vi "StartCANEngine.vi"(8 "error in (no error)":errorcluster, 10 "Buses":string[](array[string]), 11 "SmartBench in":refnum<class "SmartBench.lvclass">) -> (0 "error out":errorcluster, 3 "SmartBench out":refnum<class "SmartBench.lvclass">)   [LabVIEW 2024, in "SmartBench.lvclass"]
uses:
  SmartBench.lvclass
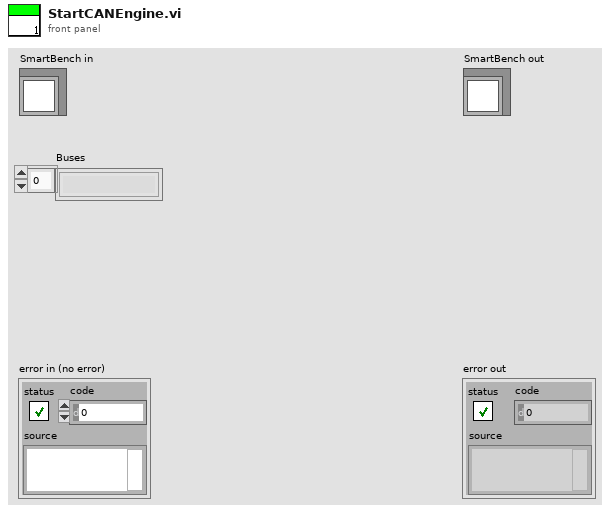
[diagram p1: front panel]
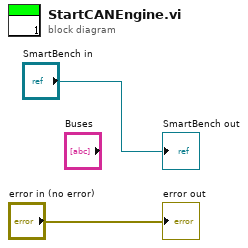
[diagram p0: block diagram]
diagram:
  "error out" <- "error in (no error)"
  "SmartBench out" <- "SmartBench in"
